vi "main-TestStand.vi"() -> ()   [LabVIEW 2018]
uses:
  <vilib>/Analysis/baseanly.llb/Mean (DBL).vi
  <vilib>/DAQmx/write.llb/DAQmx Write (Analog DBL 1Chan 1Samp).vi
  <vilib>/DAQmx/create/channels.llb/DAQmx Create Channel (AO-Voltage-Basic).vi
  <vilib>/DAQmx/miscellaneous.llb/DAQmx Fill In Error Info.vi
  <vilib>/Analysis/NI_AALBase.lvlib
panel:
  in  "dimension size":i32
  in  "milliseconds to wait":u32
  out "Ereg Setpoint":dbl
  out "Ereg":dynamicdata(graph)
  out "Pressure Transducer":dynamicdata(graph)
  out "Ereg Pressure":dbl
  out "Pressure Drop":dbl
  out "Actual Pressure":dbl
  in  "Target Pressure (psi) 2":dbl
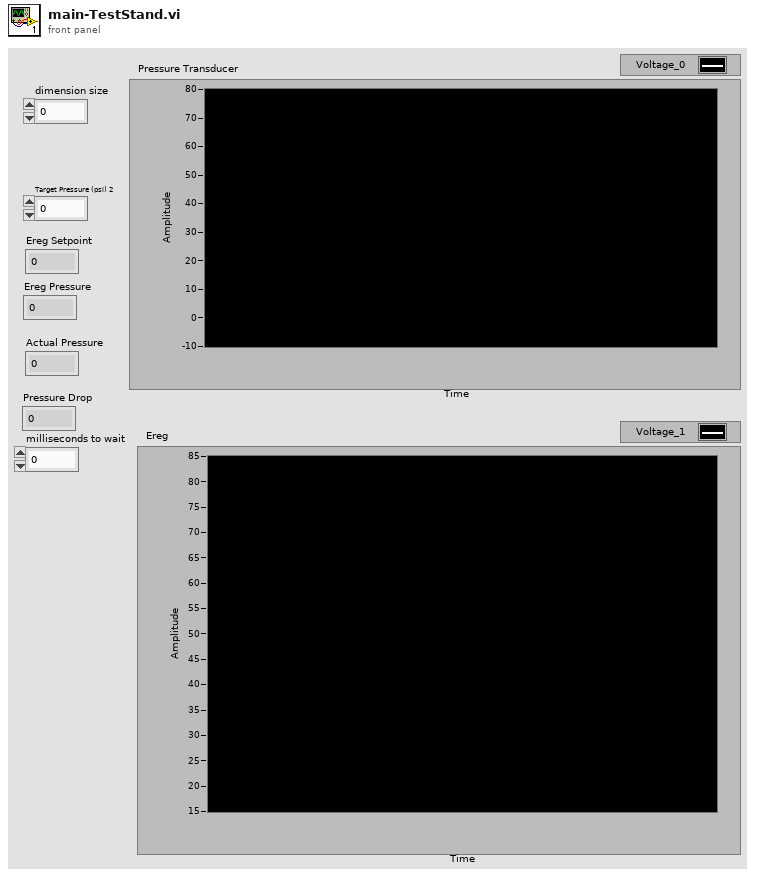
[diagram p1: front panel]
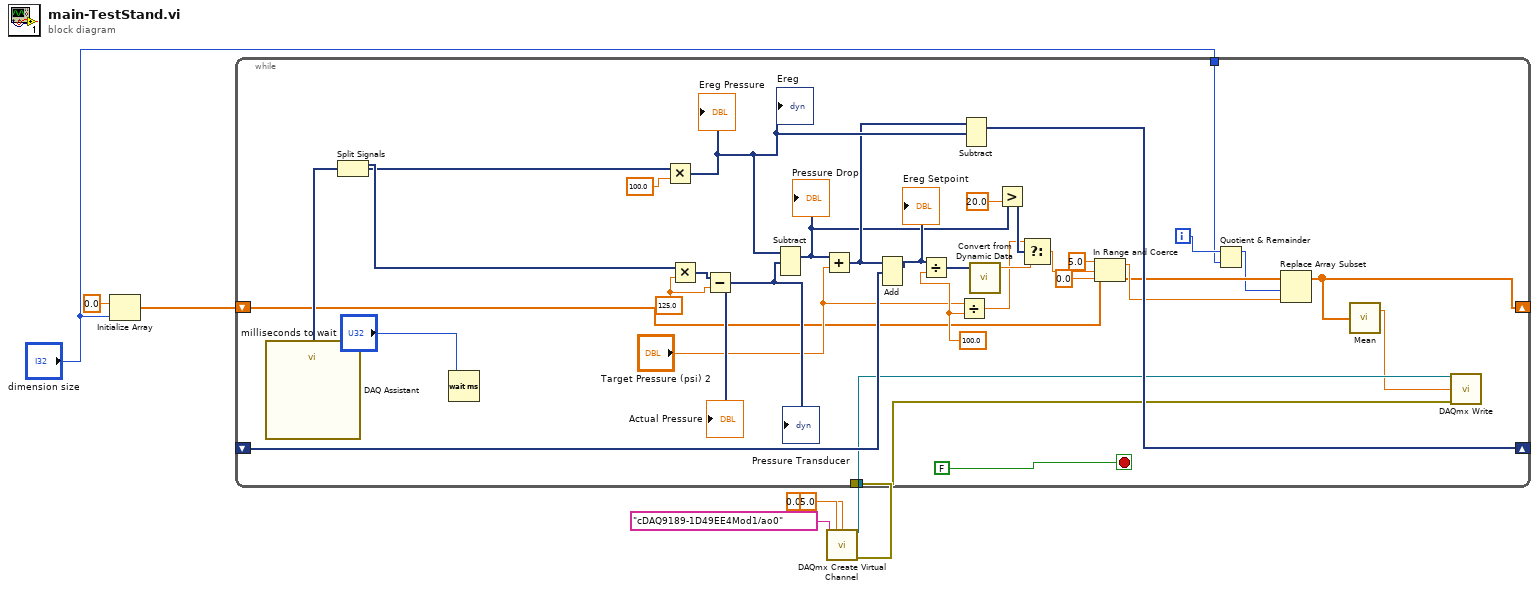
[diagram p0: block diagram]
diagram:
  n1 = Initialize Array(0.0 ("element"), "dimension size") -> (w3:dbl[])
  n2 = call-poly <vilib>:"DAQmx Create Virtual Channel.vi"("maximum value"=5.0, "minimum value"=0.0, "physical channels"=tag "cDAQ9189-1D49EE4Mod1/ao0") -> ("task out"=w5:refnum<k21>, "error out"=w4:errorcluster)  [unwired: 11 in]
  n3 = while {
    shift-right: [w29] -> _
    shift-left: _ -> [w27]
    tunnel: w5 -> [w17]
    tunnel: w4 -> [w16]
    shift-right: [w11] -> _
    shift-left: w3 -> [w14]
    tunnel: "dimension size" -> [w12]
    i -> [w13]
    stop <- FALSE stop-if-true
    w20 = 100.0 ("y")
    w39 = 125.0 ("Conversion Factor")
    n4 = call "DAQ Assistant"() -> ("data"=w34:dynamicdata)  [unwired: 16 in, 3 out]
    n5 = Split Signals(w34) -> (w33:dynamicdata, w32:dynamicdata)  [unwired: 2 in]
    n6 = Wait (ms)(milliseconds to wait="milliseconds to wait") -> ()  [unwired: 1 out]
    n7 = Multiply(x=w32, y=100.0) -> (x*y=w30:dynamicdata)
    "Ereg Pressure" <- w30
    "Ereg" <- w30
    n8 = Multiply(x=w33, y=w39) -> (x*y=w40:dynamicdata)
    n9 = Subtract(x=w40, y=w39) -> (x-y=w38:dynamicdata)
    "Actual Pressure" <- w38
    "Pressure Transducer" <- w38
    n10 = Subtract(1:w38, 2:w30) -> (0:w21:dynamicdata)  [unwired: 1 in, 1 out]
    "Pressure Drop" <- w21
    n11 = Add(x=w21, y="Target Pressure (psi) 2") -> (x+y=w28:dynamicdata)
    n12 = Add(1:w27, 2:w28) -> (0:w26:dynamicdata)  [unwired: 1 in, 1 out]
    "Ereg Setpoint" <- w26
    n13 = Divide(x=w26, y=w20) -> (x/y=w37:dynamicdata)
    n14 = Divide(x="Target Pressure (psi) 2", y=w20) -> (x/y=w18:dbl)
    n15 = Subtract(1:w30, 2:w28) -> (0:w29:dynamicdata)  [unwired: 1 in, 1 out]
    n16 = call "Convert from Dynamic Data"("Dynamic Data Type"=w37) -> ("Scalar"=w25:dbl)  [unwired: 3 in]
    n17 = Greater?(x=w21, y=20.0) -> (0:w22:dynamicdata)
    n18 = Select(t=w18, s=w22, f=w25) -> (s? t:f=w24:dbl)
    n19 = In Range and Coerce(upper limit=5.0, x=w24, lower limit=0.0) -> (coerced(x)=w15:dbl)  [unwired: 1 out]
    n20 = Quotient & Remainder(x=w13, y=w12) -> (x-y*floor(x/y)=w9:i32)  [unwired: 1 out]
    n21 = Replace Array Subset(array=w14, new element=w15, index=w9) -> (w11:dbl[])
    n22 = call-poly <vilib>:"Mean.vi"("X"=w11) -> ("mean"=w10:dbl)  [unwired: 1 out]
    n23 = call-poly <vilib>:"DAQmx Write.vi"("task/channels in"=w17, "data"=w10, "error in"=w16) -> ()  [unwired: 10 in, 3 out]
  }
